vi "post_pelletron_data.vi"(7 "error in (no error)":errorcluster, 10 "Input data":T1) -> (0 "error out":errorcluster)   [LabVIEW 2013]
uses:
  User Interface/Controls/PelletronLabview.ctl
  User Interface/Controls/Pelletron.ctl
  Sub-Polymorphic/post_pelletron.vi
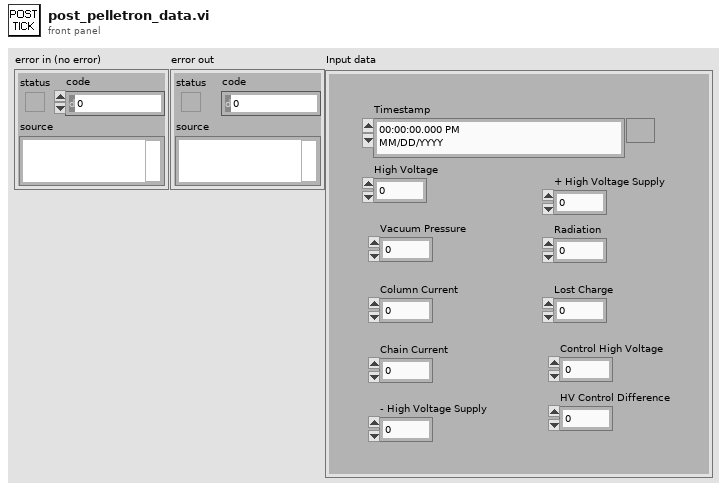
[diagram p1: front panel]
types:
  T1 = typedef "PelletronLabview.ctl" = cluster{"Timestamp":timestamp, "High Voltage":sgl, "+ High Voltage Supply":dbl, "- High Voltage Supply":dbl, "HV Control Difference":dbl, "Vacuum Pressure":sgl, "Radiation":dbl, "Column Current":sgl, "Lost Charge":dbl, "Chain Current":sgl, "Control High Voltage":dbl}
  T2 = typedef "Pelletron.ctl" = cluster{"ID":i32, "Integer Timestamp":u64, "High Voltage":sgl, "+ High Voltage Supply":sgl, "- High Voltage Supply":sgl, "HV Control Difference":sgl, "Vacuum Pressure":sgl, "Radiation":sgl, "Column Current":sgl, "Lost Charge":sgl, "Chain Current":sgl, "Control High Voltage":sgl}
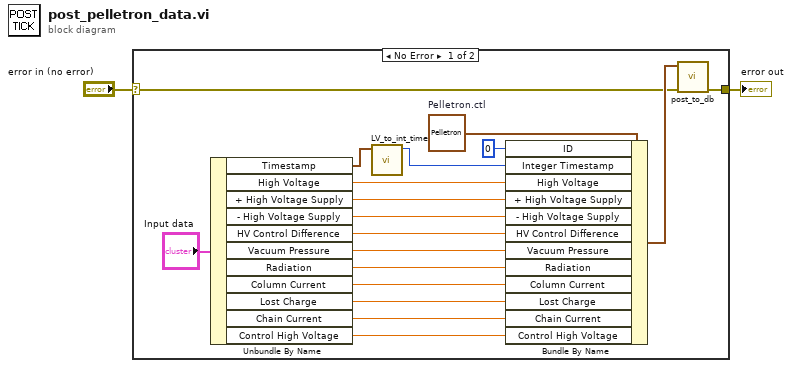
[diagram p0: block diagram]
diagram:
  n1 = case shown="No Error" "error in (no error)" {
    selector: "error in (no error)" -> [w4 w21]
    tunnel: [w3 w21] -> w1
    frame No Error {
      w20 = T2 {"ID"=0, "Integer Timestamp"=0, "High Voltage"=0.0, "+ High Voltage Supply"=0.0, "- High Voltage Supply"=0.0, "HV Control Difference"=0.0, "Vacuum Pressure"=0.0, "Radiation"=0.0, "Column Current"=0.0, "Lost Charge"=0.0, "Chain Current"=0.0, "Control High Voltage"=0.0}  # Pelletron.ctl
      n2 = Unbundle By Name("Input data") -> ("Timestamp"=w17:timestamp, "High Voltage"=w16:sgl, "+ High Voltage Supply"=w15:dbl, "- High Voltage Supply"=w14:dbl, "HV Control Difference"=w13:dbl, "Vacuum Pressure"=w12:sgl, "Radiation"=w11:dbl, "Column Current"=w10:sgl, "Lost Charge"=w9:dbl, "Chain Current"=w8:sgl, "Control High Voltage"=w7:dbl)
      n3 = call "LV_to_int_time.vi"("Time Stamp"=w17) -> ("Integer Time"=w19:i64)  [unwired: 8 in, 1 out]
      n4 = Bundle By Name(cluster=w20, "ID"=0, "Integer Timestamp"=w19, "High Voltage"=w16, "+ High Voltage Supply"=w15, "- High Voltage Supply"=w14, "HV Control Difference"=w13, "Vacuum Pressure"=w12, "Radiation"=w11, "Column Current"=w10, "Lost Charge"=w9, "Chain Current"=w8, "Control High Voltage"=w7) -> (w5:T2)
      n5 = call-poly "post_to_db.vi"("error in (no error)"=w4, "Pelletron Data"=w5) -> ("error out"=w3:errorcluster)  [unwired: 9 in]
    }
    frame Error {
    }
  }
  "error out" <- w1
